vi "set_sample_dwell_time.vi"(8 "error in (no error)":errorcluster, 10 "sample dwell time":dbl[unit], 11 "GenericWriteSignals.lvclass in":refnum<class "SignalWriterMH110203USBStepperMotor.lvclass">) -> (0 "error out":errorcluster, 3 "GenericWriteSignals.lvclass out":refnum<class "SignalWriterMH110203USBStepperMotor.lvclass">)   [LabVIEW 2010, in "SignalWriterMH110203USBStepperMotor.lvclass"]
uses:
  SignalWriterMH110203USBStepperMotor.lvclass
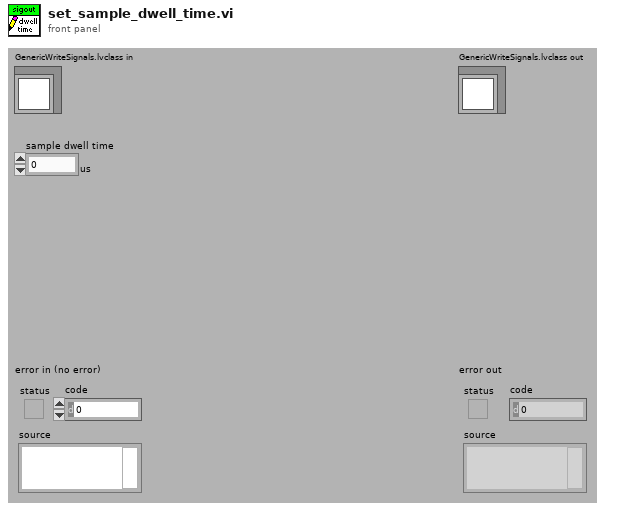
[diagram p1: front panel]
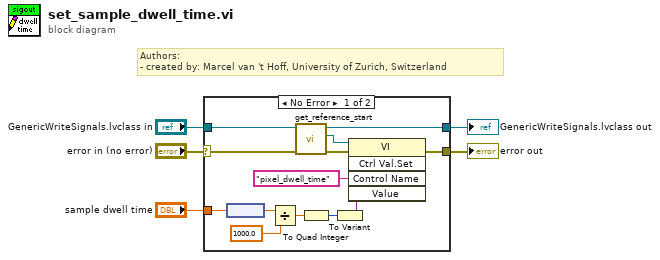
[diagram p0: block diagram]
diagram:
  # "Authors: \n- created by: Marcel van 't Hoff, University of Zurich, Switzerland"
  n1 = case shown="No Error" "error in (no error)" {
    selector: "error in (no error)" -> [w12 w20]
    tunnel: [w11 w20] -> w3
    tunnel: "GenericWriteSignals.lvclass in" -> [w14 w19]
    tunnel: [w13 w19] -> w2
    tunnel: "sample dwell time" -> [w10 _]
    frame No Error {
      n2 = node(w10) -> (w8:dbl)
      n3 = Divide(x=w8, y=1000.0) -> (x/y=w7:dbl)
      n4 = call-dynamic "get_reference_start.vi"("error in (no error)"=w12, "SignalWriterMH110203USBStepperMotor in"=w14) -> ("error out"=w17:errorcluster, "vi reference"=w18:refnum<vi>, "SignalWriterMH110203USBStepperMotor out"=w13:refnum<class "SignalWriterMH110203USBStepperMotor.lvclass">)  [unwired: 7 in]
      n5 = To Quad Integer(1:w7) -> (0:w9:i64)
      n6 = To Variant(anything=w9) -> (Variant=w16:variant)
      n7 = invoke class="VI" method="Ctrl Val.Set"(reference=w18, error in=w17, "Control Name"="pixel_dwell_time", "Value"=w16) -> (error out=w11:errorcluster)  [unwired: 1 in, 4 out]
    }
    frame Error {
    }
  }
  "error out" <- w3
  "GenericWriteSignals.lvclass out" <- w2
